vi "to_json.vi"(8 "error in":errorcluster, 11 "ts.iso8601 in":refnum<class "ts.iso8601.lvclass">) -> (0 "error out":errorcluster, 2 "json":string, 3 "ts.iso8601 out":refnum<class "ts.iso8601.lvclass">, 4 "Not Default":bool)   [LabVIEW 2020, in "ts.iso8601.lvclass"]
uses:
  ts.iso8601.lvclass
  ts.iso8601.lvclass/ts.iso8601.ctl
  6bf8de66-28e8-4e60-b919-903522d86b70.vi
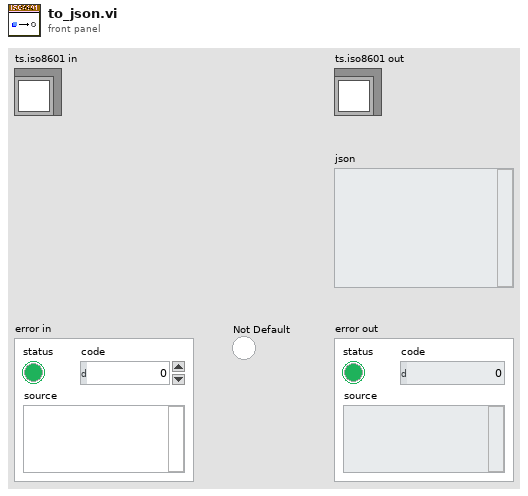
[diagram p1: front panel]
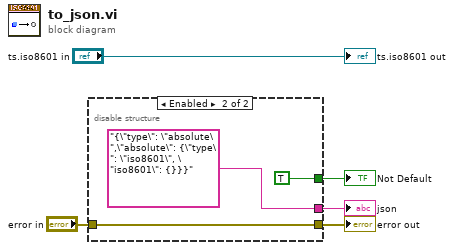
[diagram p0: block diagram]
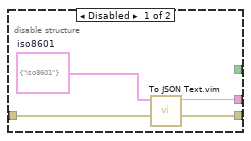
[diagram p2: hidden frame]
diagram:
  n1 = disable-structure shown="Enabled" {
    disable-tunnel: [w9 "{\"type\": \"absolute\",\"absolute\": {\"type\": \"iso8601\", \"iso8601\": {}}}"] -> w4
    disable-tunnel: [w8 w11] -> w3
    disable-tunnel: "error in" -> [w7 w11]
    disable-tunnel: [_ TRUE ("Not Default")] -> w1
    frame Disabled {
      w6 = cluster{"type":string} {"type"="iso8601"}  # iso8601
      n2 = call "To JSON Text.vim"("error in (no error)"=w7, "Anything"=w6) -> ("error out"=w8:errorcluster, "<JSON>"=w9:string)  [unwired: 8 in]
    }
    frame Enabled {
    }
  }
  "error out" <- w3
  "json" <- w4
  "Not Default" <- w1
  "ts.iso8601 out" <- "ts.iso8601 in"
